vi "cRIO Read Module EEPROM.vi"(8 "error in":errorcluster, 11 "Session in":refnum<k21>="localhost") -> (0 "error out":errorcluster, 2 "EEPROM Data":string, 3 "Session out":refnum<k21>="localhost")   [LabVIEW 2015, in "RT Management.lvlib" / "Module Detection.lvclass"]
uses:
  Module Detection.lvclass
  <vilib>/rvi/interface/nirviCloseFPGA/nirviCloseFPGA.xnode
  <vilib>/rvi/interface/nirviMethod/nirviMethod.xnode
  <vilib>/FPGAPlugInAG/Dynamic/niLvFpga_Close_Dynamic.vi
  <vilib>/rvi/interface/nirviReadWriteControl/nirviReadWriteControl.xnode
  NiFpgaLv.dll
  <vilib>/Utility/error.llb/Error Cluster From Error Code.vi
  <vilib>/rvi/interface/Simulation/niFpgaSimulationCallBeginRW.vi
  <vilib>/rvi/errors/niLvFpgaAdjustHostInterfaceError.vi
  <vilib>/FPGAPlugInAG/Dynamic/niLvFpga_Run_Dynamic.vi
  RT Management/RT Management.lvclass
panel:
  in  "Module":u16
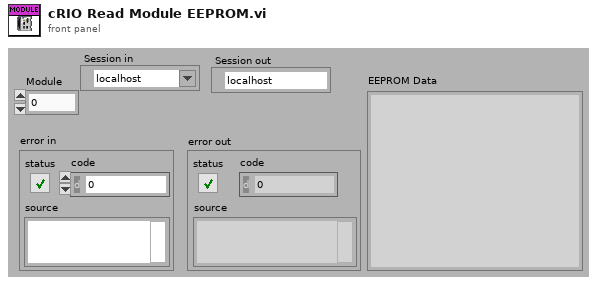
[diagram p1: front panel]
types:
  T1 = typedef "RT Management.lvlib/Device.lvclass/NetworkDevice.ctl" = cluster{"System Hardware Reference":refnum<k20>, "Device Information":T2, "Network Adapter Settings":T3[]}
  T2 = typedef "RT Management.lvlib/Device.lvclass/DeviceInformation.ctl" = cluster{"Resource":string, "Vendor Name":string, "Product Name":string, "Product ID":u32, "Serial Number":string, "Device Class":string, "System Start Time":timestamp, "Current Time":timestamp, "Time Zone":string, "Firmware Revision":string, "Image Title":string, "Image Version":string, "System Status":string}
  T3 = typedef "RT Management.lvlib/Device.lvclass/NetworkAdapterSettings.ctl" = cluster{"IP Address":string, "MAC Address":string, "IP Address Request Mode":u32, "SubnetMask":string, "Gateway":string, "DNS Server":string, "Adapter Mode":u32, "Adapter Type":u32, "Is Primary Adapter":bool}
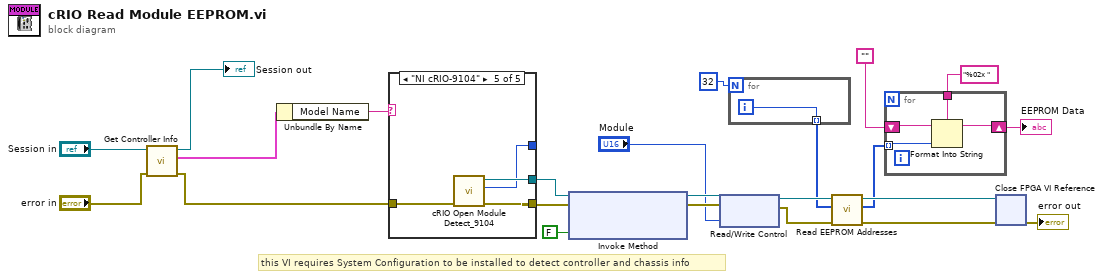
[diagram p0: block diagram]
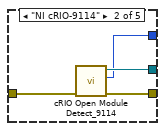
[diagram p3: hidden frame]
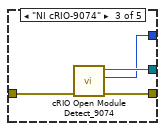
[diagram p4: hidden frame]
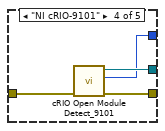
[diagram p5: hidden frame]
diagram:
  # "this VI requires System Configuration to be installed to detect controller and chassis info"
  n1 = call "Get Controller Info.vi"("error in"="error in", "Session in"="Session in") -> ("error out"=w4:errorcluster, "Network Device"=w3:T1, "Session out"=→"Session out":refnum<k21>)  [unwired: 7 in]
  n2 = Unbundle By Name(w3) -> ("Model Name"=w19:string)
  n3 = case shown="\"NI cRIO-9104\"" w19 {
    tunnel: w4 -> [w24 w28 w31 w35 w39]
    tunnel: [_ w27 w30 w34 w38] -> w20
    tunnel: [w24 w26 w32 w36 w40] -> w21
    tunnel: [_ w25 w29 w33 w37] -> _
    frame "<Undefined>", Default {
    }
    frame "NI cRIO-9114" {
      n4 = call "cRIO Open Module Detect_9114.vi"("error in (no error)"=w28) -> ("error out"=w26:errorcluster, "slots"=w25:i32, "Refnum out"=w27:refnum<k20>)  [unwired: 8 in]
    }
    frame "NI cRIO-9074" {
      n5 = call "cRIO Open Module Detect_9074.vi"("error in (no error)"=w31) -> ("error out"=w32:errorcluster, "slots"=w29:i32, "Refnum out"=w30:refnum<k20>)  [unwired: 8 in]
    }
    frame "NI cRIO-9101" {
      n6 = call "cRIO Open Module Detect_9101.vi"("error in (no error)"=w35) -> ("error out"=w36:errorcluster, "slots"=w33:i32, "Refnum out"=w34:refnum<k20>)  [unwired: 8 in]
    }
    frame "NI cRIO-9104" {
      n7 = call "cRIO Open Module Detect_9104.vi"("error in (no error)"=w39) -> ("error out"=w40:errorcluster, "slots"=w37:i32, "Refnum out"=w38:refnum<k20>)  [unwired: 8 in]
    }
  }
  n8 = xnode "Invoke Method"("FPGA VI Reference In"=w20, "error in"=w21, "Wait Until Done (F)"=FALSE) -> ("FPGA VI Reference Out"=w18:refnum<k20>, "error out"=w17:errorcluster)
  n9 = xnode "Read/Write Control"("FPGA VI Reference In"=w18, "error in"=w17, "Module"="Module") -> ("FPGA VI Reference Out"=w14:refnum<k20>, "error out"=w15:errorcluster)
  n10 = for {
    N: 32 -> [_]
    tunnel: [w41] -> w12 mode=indexing
    i -> [w41]
  }
  n11 = call "Read EEPROM Addresses.vi"("error in (no error)"=w15, "Addresses"=w12, "Refnum in"=w14) -> ("error out"=w13:errorcluster, "Data"=w6:u8[], "Refnum out"=w10:refnum<k20>)  [unwired: 6 in]
  n12 = for {
    tunnel: "%02x " ("format string") -> [w45]
    tunnel: w6 -> [w44] mode=indexing
    shift-right: [w43] -> w7
    shift-left: "" -> [w42]
    n13 = Format Into String(format string=w45, initial string=w42, w44) -> (resulting string=w43:string)  [unwired: 1 in, 1 out]
  }
  "EEPROM Data" <- w7
  n14 = xnode "Close FPGA VI Reference"("FPGA VI Reference In"=w10, "error in"=w13) -> ("error out"=→"error out":errorcluster)
